vi "Test Double Click.vi"() -> ()   [LabVIEW 2019]
panel:
  out "Table Control 2":string[][](table)
  out "Table Control":string[][](table)
  in  "file path (dialog if empty)":path=path "C:/Users/CHIAM KOK THIAM/Downloads/tdk/check double click/wfm"
  out "Peak Indexes":i32[](array[numeric])
  out "Waveform Graph 2":dbl[](graph)
  out "Waveform Graph":waveform(dbl)(graph)
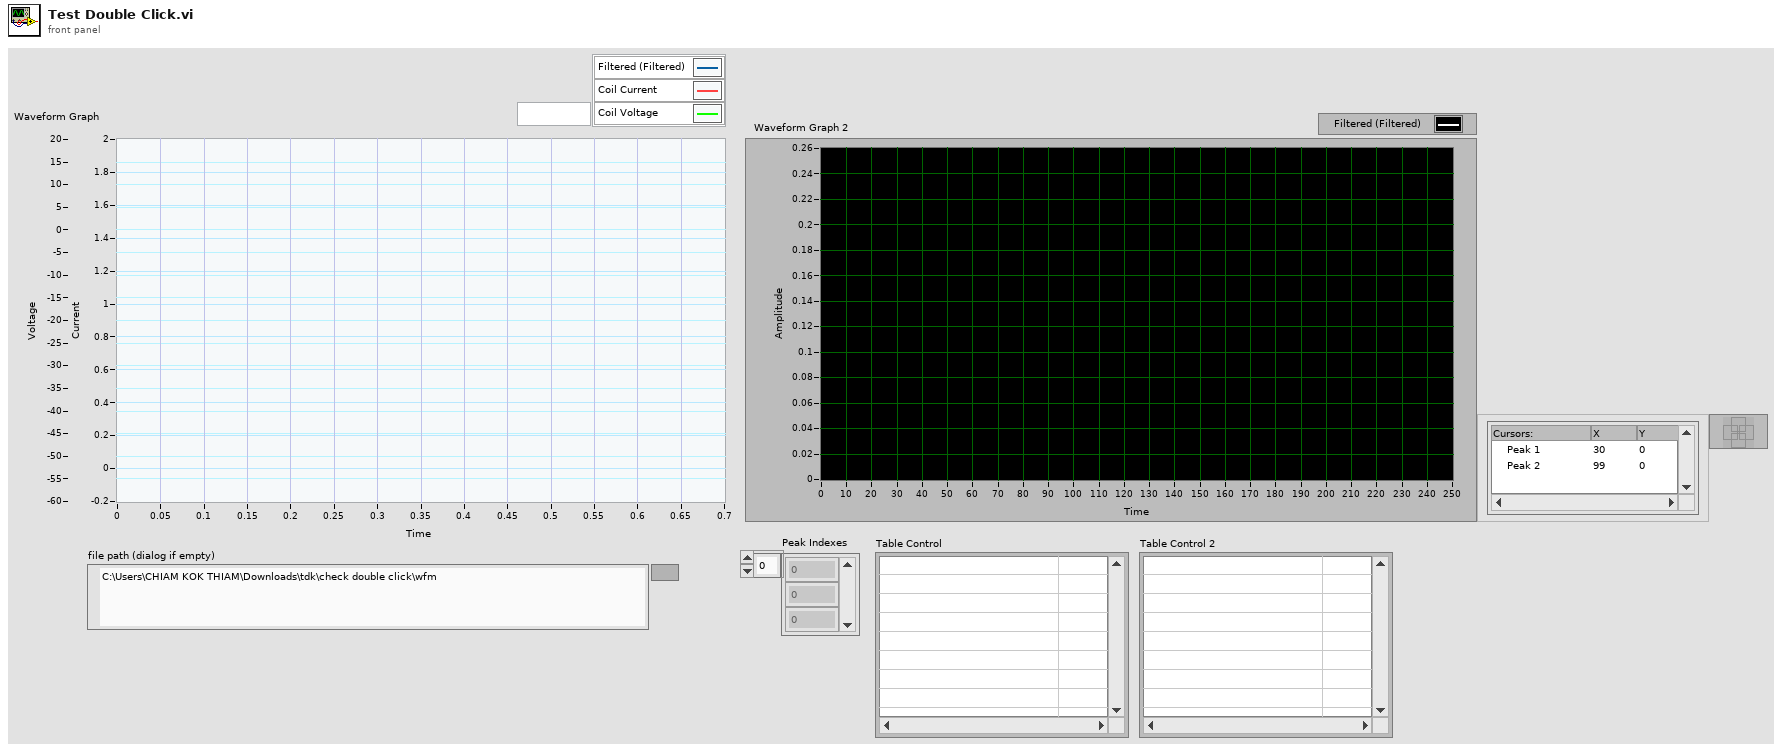
[diagram p1: front panel]
types:
  T1 = cluster{"Name":string, "Color":u32, "Style":u8, "Point Style":u8, "Name Visible":bool, "Allow Drag":bool, "Cursor Mode":u32, "Plot":i32, "Index":i32, "Position":cluster{"X":dbl, "Y":dbl}, "X Scale":u32, "Y Scale":u32, "Watch Plots":i32[], "Watch All Plots":bool, "Plot Area":i32, "Label Offset":cluster{"X":dbl, "Y":dbl}}
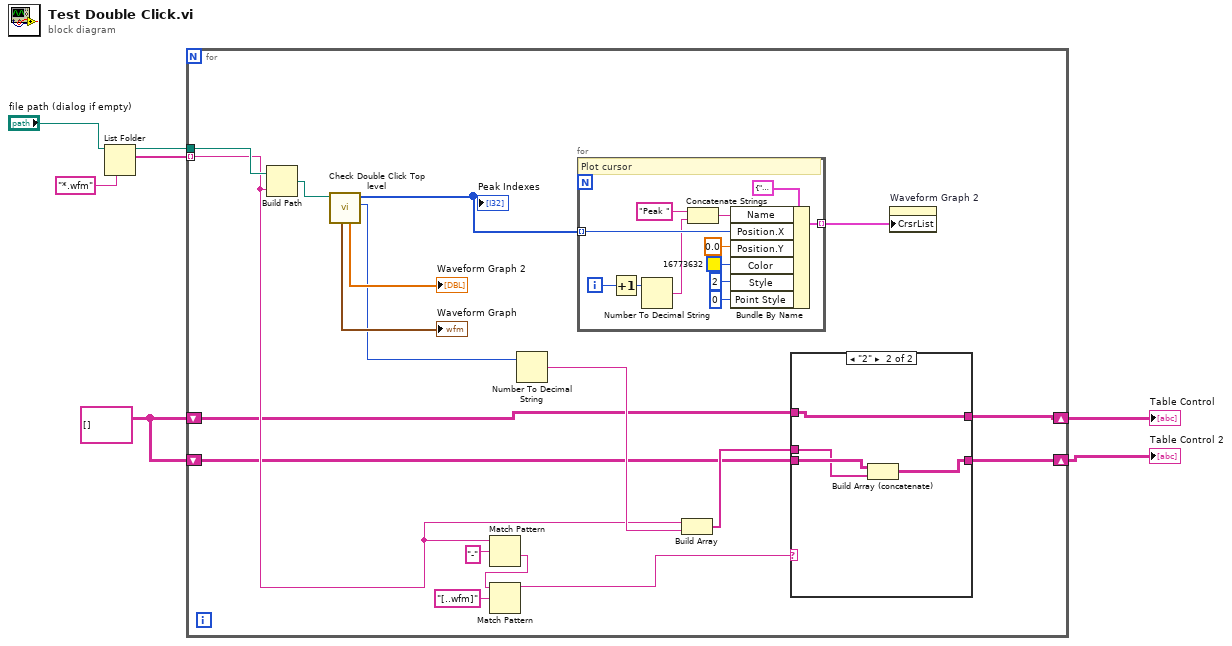
[diagram p0: block diagram]
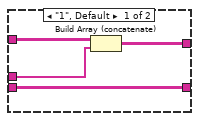
[diagram p2: hidden frame]
diagram:
  w3 = string[][] []
  n1 = List Folder(path="file path (dialog if empty)", pattern="*.wfm") -> (path out=w5:path, filenames=w6:string[])  [unwired: 2 in, 2 out]
  n2 = for {
    tunnel: w6 -> [w16] mode=indexing
    tunnel: w5 -> [w21]
    shift-right: [w13] -> w2
    shift-left: w3 -> [w12]
    shift-right: [w10] -> w1
    shift-left: w3 -> [w11]
    n3 = Build Path(base path=w21, name or relative path=w16) -> (appended path=w20:path)
    n4 = call "Check Double Click Top level.vi"("path"=w20) -> ("Number of Peaks"=w19:i32, "Peak Indexes"=w24:i32[], "Y"=→"Waveform Graph 2":dbl[], "Waveform Graph"=→"Waveform Graph":waveform(dbl))  [unwired: 6 in, 1 out]
    "Peak Indexes" <- w24
    n5 = Match Pattern(string=w16, regular expression="-") -> (after substring=w15:string)  [unwired: 1 in, 3 out]
    n6 = Match Pattern(string=w15, regular expression="[..wfm]") -> (before substring=w8:string)  [unwired: 1 in, 3 out]
    n7 = Number To Decimal String(number=w19) -> (decimal integer string=w18:string)  [unwired: 1 in]
    n8 = for {
      tunnel: w24 -> [w42] mode=indexing
      tunnel: [w43] -> w23 mode=indexing
      i -> [w45]
      # "Plot cursor"
      n9 = Increment(x=w45) -> (x+1=w44:i32)
      n10 = Number To Decimal String(number=w44) -> (decimal integer string=w39:string)  [unwired: 1 in]
      n11 = Concatenate Strings("Peak " ("Name"), w39) -> (w41:string)
      n12 = Bundle By Name(cluster=T1 {"Name"="", "Color"=0, "Style"=0, "Point Style"=0, "Name Visible"=FALSE, "Allow Drag"=FALSE, "Cursor Mode"=0, "Plot"=0, "Index"=0, "Position"={"X"=0.0, "Y"=0.0}, "X Scale"=0, "Y Scale"=0, "Watch Plots"=[], "Watch All Plots"=FALSE, "Plot Area"=0, "Label Offset"={"X"=0.0, "Y"=0.0}}, "Name"=w41, "Position.X"=w42, "Position.Y"=0.0 ("Position.X"), "Color"=u32 16773632, "Style"=u8 2, "Point Style"=u8 0) -> (w43:T1)
    }
    n13 = Build Array(w16, w18) -> (w14:string[])
    n14 = case shown="\"2\"" w8 {
      tunnel: w14 -> [w29 w32]
      tunnel: [w28 w30] -> w13
      tunnel: w12 -> [w27 w30]
      tunnel: w11 -> [w26 w33]
      tunnel: [w26 w31] -> w10
      frame "1", Default {
        n15 = Build Array (concatenate)(w27, w29) -> (w28:string[][])
      }
      frame "2" {
        n16 = Build Array (concatenate)(w33, w32) -> (w31:string[][])
      }
    }
    n17 = property on="Waveform Graph 2" class="WFGraph (strict)"("CrsrList"=w23) -> ()  [unwired: 2 in, 2 out]
  }
  "Table Control" <- w2
  "Table Control 2" <- w1
